vi "Set Default Case By Frame Name.vi"(8 "error in (no error)":errorcluster, 10 "Frame Name":string, 11 "CaseStructure in":refnum<vi>) -> (0 "error out":errorcluster, 3 "CaseStructure out":refnum<vi>)   [LabVIEW 2019, in "gRPC Template Creation Utility.lvlib"]
uses:
  gRPC Template Creation Utility.lvlib
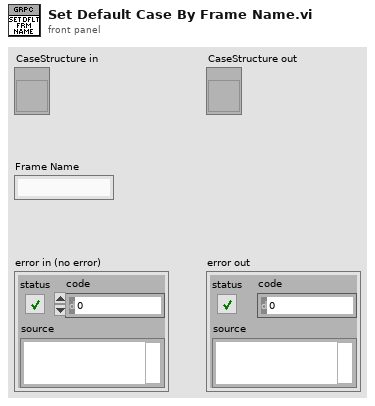
[diagram p1: front panel]
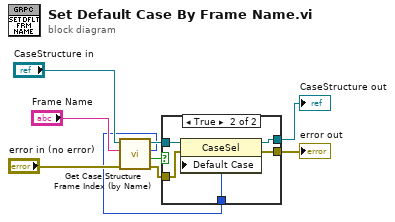
[diagram p0: block diagram]
diagram:
  n1 = call "Get Case Structure Frame Index (by Name).vi"("error in (no error)"="error in (no error)", "element"="Frame Name", "CaseStructure in"="CaseStructure in") -> ("error out"=w2:errorcluster, "Found?"=w6:bool, "Frame Index"=w1:i32, "CaseStructure out"=w7:refnum<vi>)  [unwired: 5 in]
  n2 = case shown="True" w6 {
    tunnel: [w11 w16] -> w9
    tunnel: w7 -> [w11 w15]
    tunnel: [w10 w14] -> w3
    tunnel: w2 -> [w10 w13]
    tunnel: w1 -> [_ w12]
    frame False {
    }
    frame True {
      n3 = property class="CaseSel"(reference=w15, error in=w13, "Default Case"=w12) -> (reference out=w16:refnum<vi>, error out=w14:errorcluster)
    }
  }
  "error out" <- w3
  "CaseStructure out" <- w9
